vi "Test.vi"() -> ()   [LabVIEW 2018, in "Application.lvlib" / "Store.lvclass"]
uses:
  Store.lvclass
  Store.lvclass/Store.ctl
  Dictionary Class/Dictionary.lvclass/Dictionary.ctl
  Get Dictionary.vi
  Add.vi/e194419b-6248-448c-bfd0-3bb9f5219d49.vi
  Key-Value To Packet Data.vi
  Variant to Packed String.vi
  Get All.vi/1b7bc760-b481-47a7-9710-96281ada8069.vi
  Packed String to Variant.vi
  Dictionary Class/VIs/Get Data DVR.vi
  Dictionary Class/Dictionary.lvclass
panel:
  out "size(s) 2":i32
  out "size(s)":i32
  out "Values":variant[](array[variant])
  out "Keys":variant[](array[variant])
  out "Value":variant
  out "x-y 2":dbl format="%^#_6e"
  out "x-y":dbl format="%^#_6e"
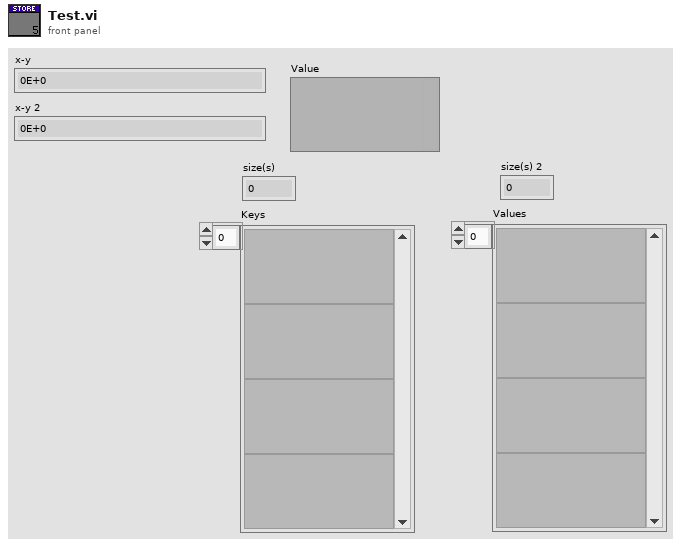
[diagram p1: front panel]
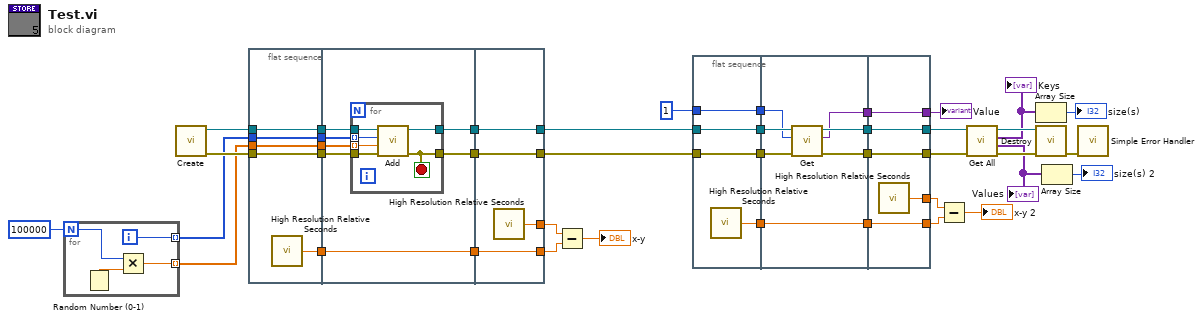
[diagram p0: block diagram]
diagram:
  n1 = for {
    N: 100000 -> [w44]
    tunnel: [w42] -> w29 mode=indexing
    tunnel: [w41] -> w9 mode=indexing
    i -> [w41]
    n2 = Random Number (0-1)() -> (number: 0 to 1=w43:dbl)
    n3 = Multiply(x=w44, y=w43) -> (x*y=w42:dbl)
  }
  n4 = call "Create.vi"() -> ("error out"=w30:errorcluster, "Store out"=w31:refnum<class "Store.lvclass">)  [unwired: 10 in]
  n5 = flat-sequence {
    tunnel: w9 -> [w46]
    tunnel: w29 -> [w47]
    tunnel: w31 -> [w48]
    tunnel: w30 -> [w49]
    tunnel: [w49] -> w39
    tunnel: [w48] -> w38
    tunnel: [w47] -> w37
    tunnel: [w46] -> w36
    tunnel: [w45] -> w35
    tunnel: w39 -> [w56]
    tunnel: w38 -> [w55]
    tunnel: w37 -> [w54]
    tunnel: w36 -> [w53]
    tunnel: [w52] -> w34
    tunnel: [w51] -> w33
    tunnel: [w50] -> w32
    tunnel: w35 -> [w50]
    tunnel: [w65] -> w23
    tunnel: [w66] -> w24
    tunnel: w34 -> [w66]
    tunnel: w33 -> [w65]
    tunnel: [w64] -> w26
    tunnel: w32 -> [w64]
    tunnel: [w63] -> w27
    frame #0 {
      n6 = call <vilib>:"High Resolution Relative Seconds.vi"() -> ("relative seconds"=w45:dbl)
    }
    frame #1 {
      n7 = for {
        tunnel: w56 -> [w61]
        tunnel: w55 -> [w62]
        tunnel: w54 -> [w57] mode=indexing
        tunnel: w53 -> [w58] mode=indexing
        tunnel: [w60] -> w52
        tunnel: [w59] -> w51
        stop <- w59 stop-if-true
        n8 = call "Add.vi"("error in (no error)"=w61, "Value"=w57, "Key"=w58, "Store in"=w62) -> ("error out"=w59:errorcluster, "Store out"=w60:refnum<class "Store.lvclass">)  [unwired: 5 in, 1 out]
      }
    }
    frame #2 {
      n9 = call <vilib>:"High Resolution Relative Seconds.vi"() -> ("relative seconds"=w63:dbl)
    }
  }
  n10 = Subtract(x=w27, y=w26) -> (x-y=→"x-y":dbl)
  n11 = flat-sequence {
    tunnel: w23 -> [w69]
    tunnel: w24 -> [w70]
    tunnel: [w70] -> w22
    tunnel: [w69] -> w21
    tunnel: [w68] -> w20
    tunnel: 1 -> [w67]
    tunnel: [w67] -> w15
    tunnel: w22 -> [w77]
    tunnel: w21 -> [w76]
    tunnel: w20 -> [w73]
    tunnel: [w75] -> w19
    tunnel: [w74] -> w18
    tunnel: [w73] -> w17
    tunnel: w15 -> [w72]
    tunnel: [w71] -> w11
    tunnel: [w80] -> w12
    tunnel: [w81] -> w8
    tunnel: [w82] -> w7
    tunnel: w19 -> [w82]
    tunnel: w18 -> [w81]
    tunnel: w17 -> [w80]
    tunnel: [w79] -> w13
    tunnel: w11 -> [w78]
    tunnel: [w78] -> w10
    frame #0 {
      n12 = call <vilib>:"High Resolution Relative Seconds.vi"() -> ("relative seconds"=w68:dbl)
    }
    frame #1 {
      n13 = call "Get.vi"("error in (no error)"=w76, "Key"=w72, "Store in"=w77) -> ("error out"=w75:errorcluster, "Value"=w71:variant, "Store out"=w74:refnum<class "Store.lvclass">)  [unwired: 5 in, 1 out]
    }
    frame #2 {
      n14 = call <vilib>:"High Resolution Relative Seconds.vi"() -> ("relative seconds"=w79:dbl)
    }
  }
  n15 = Subtract(x=w13, y=w12) -> (x-y=→"x-y 2":dbl)
  n16 = call "Get All.vi"("error in (no error)"=w7, "Store in"=w8) -> ("error out"=w5:errorcluster, "Values"=w4:variant[], "Keys"=w3:variant[], "Store out"=w6:refnum<class "Store.lvclass">)  [unwired: 6 in]
  "Keys" <- w3
  "Values" <- w4
  n17 = Array Size(array=w3) -> (size(s)=→"size(s)":i32)
  n18 = call "Destroy.vi"("error in (no error)"=w5, "Store in"=w6) -> ("error out"=w28:errorcluster)  [unwired: 9 in]
  n19 = Array Size(array=w4) -> (size(s)=→"size(s) 2":i32)
  n20 = call <vilib>:"Simple Error Handler.vi"("error in (no error)"=w28) -> ()  [unwired: 4 in, 5 out]
  "Value" <- w10
